vi "Format Search Params.vi"(4 "Search Items":T1[](array[typedef])) -> (1 "URL Param String":string, 2 "Raw Param String":string)   [LabVIEW 2024, in "ETL API.lvlib"]
uses:
  ETL API.lvlib
  ETL Search Element.ctl
  <vilib>/addons/_JKI.lib/REST Client/classes/REST Client/REST Client.lvclass
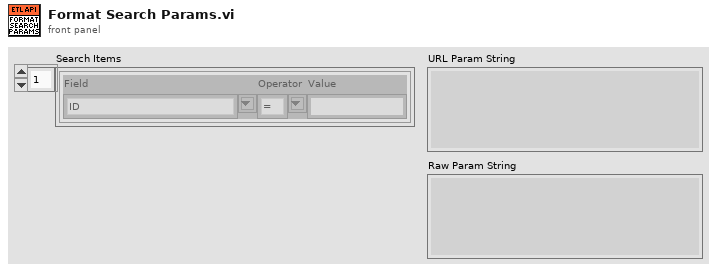
[diagram p1: front panel]
types:
  T1 = typedef "ETL API.lvlib/ETL Search Element.ctl" = cluster{"Field":string, "Operator":string, "Value":string}
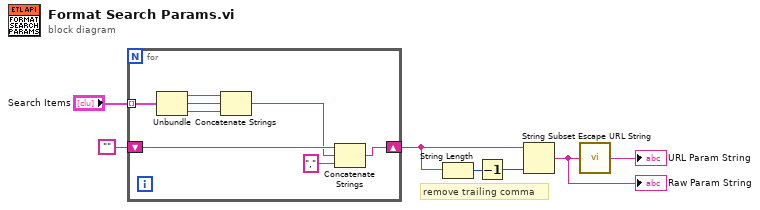
[diagram p0: block diagram]
diagram:
  # "remove trailing comma"
  n1 = for {
    tunnel: "Search Items" -> [w15] mode=indexing
    shift-right: [w11] -> w7
    shift-left: "" -> [w13]
    n2 = Unbundle(w15) -> ("Field"=w14:string, "Operator"=w10:string, "Value"=w9:string)
    n3 = Concatenate Strings(w14, w10, w9) -> (w8:string)
    n4 = Concatenate Strings(w13, w8, "," ("string")) -> (w11:string)
  }
  n5 = String Length(string=w7) -> (length=w6:i32)
  n6 = Decrement(x=w6) -> (x-1=w5:i32)
  n7 = String Subset(string=w7, length (rest)=w5) -> (substring=w1:string)  [unwired: 1 in]
  "Raw Param String" <- w1
  n8 = call <vilib>:"Escape URL String.vi"("Unescaped URL string in"=w1) -> ("Escaped URL string out"=→"URL Param String":string)
